vi "test_OneSessTwoPinOneInstrOneSiteReservation_CallNiDcPowerGetConnectionsNPinsMConnections_ReturnsThreeConnections.vi"(8 "error in":errorcluster) -> (0 "error out":errorcluster, 2 "result":string, 3 "pass":bool)   [LabVIEW 2020, in "MeasurementServerTests.lvlib"]
uses:
  MeasurementServerTests.lvlib
  Runtime/Measurements/Measurement Plugin Session Management V1/Session Reservation/Connection.ctl
  Runtime/Measurements/Measurement Plugin Session Management V1/Session Reservation/Session Reservation.lvclass
  03fc85e1-696b-4ece-a78b-f41470766ac0.vi
  Runtime/Sessions/niDCPower Sessions/niDCPower Sessions.lvlib
  Runtime/Sessions/niDCPower Sessions/Connection with Session.ctl
  a536e905-e99b-4ce6-9f7b-add65bd26abc.vi
  Runtime/Sessions/niDCPower Sessions/Get Connections - NPin MConn.vi
  f2d0f46c-20cf-4e81-b3a3-5c4fc317eda1.vi
  e27c92da-164e-4bbf-942b-5ac64848be94.vi
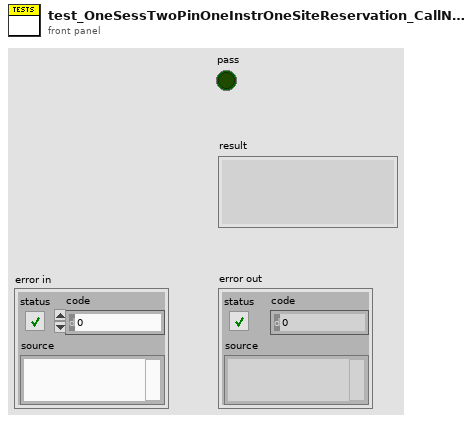
[diagram p1: front panel]
types:
  T1 = typedef "Measurement Plugin Session Management V1.lvlib/Session Reservation.lvclass/Connection.ctl" = cluster{"pin or relay name":string, "site":i32, "instrument type id":string, "channel":string}
  T2 = typedef "niDCPower Sessions.lvlib/Connection with Session.ctl" = cluster{"connection":T1, "session":refnum<k15>}
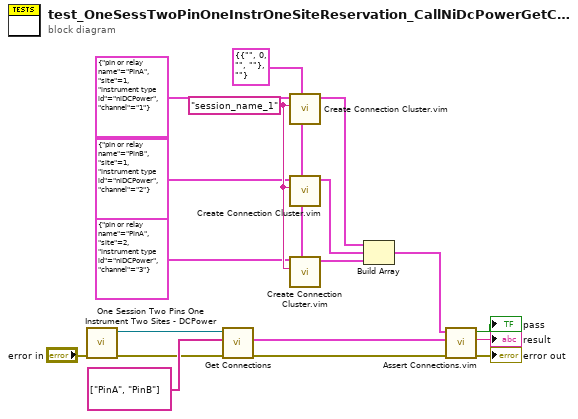
[diagram p0: block diagram]
diagram:
  w8 = T2 {"connection"={"pin or relay name"="", "site"=0, "instrument type id"="", "channel"=""}, "session"=""} ("niDCPower connection")
  w9 = "session_name_1" ("session in")
  n1 = call "One Session Two Pins One Instrument Two Sites - DCPower.vi"("error in"="error in") -> ("error out"=w4:errorcluster, "session reservation out"=w3:refnum<class "Session Reservation.lvclass">)  [unwired: 9 in]
  n2 = call-poly "Get Connections.vi"("error in"=w4, "pin or relay names"=string[] ["PinA", "PinB"], "session reservation in"=w3) -> ("error out"=w2:errorcluster, "connections"=w18:T2[])  [unwired: 6 in, 1 out]
  n3 = call "Create Connection Cluster.vim"("connection type"=w8, "session in"=w9, "hardware independent connection in"=T1 {"pin or relay name"="PinA", "site"=1, "instrument type id"="niDCPower", "channel"="1"} ("connection")) -> ("connection out"=w13:T2)  [unwired: 8 in]
  n4 = call "Create Connection Cluster.vim"("connection type"=w8, "session in"=w9, "hardware independent connection in"=T1 {"pin or relay name"="PinB", "site"=1, "instrument type id"="niDCPower", "channel"="2"} ("connection")) -> ("connection out"=w12:T2)  [unwired: 8 in]
  n5 = call "Create Connection Cluster.vim"("connection type"=w8, "session in"=w9, "hardware independent connection in"=T1 {"pin or relay name"="PinA", "site"=2, "instrument type id"="niDCPower", "channel"="3"} ("connection")) -> ("connection out"=w7:T2)  [unwired: 8 in]
  n6 = Build Array(w13, w12, w7) -> (w11:T2[])
  n7 = call "Assert Connections.vim"("error in"=w2, "actual connections"=w18, "expected connections"=w11) -> ("error out"=→"error out":errorcluster, "result"=→"result":string, "pass"=→"pass":bool)  [unwired: 6 in]
